vi "Test Case, Table Cell Color.vi"() -> ()   [LabVIEW 2010]
panel:
  in  "dst col":i32=3
  in  "dst row":i32=3
  in  "n rows":i32=5
  in  "error in":errorcluster
  out "error out":errorcluster
  in  "Dst":string[][](table)
  in  "Src":string[][](table)=[["", "", ""], ["", "", ""], ["", "", ""]]
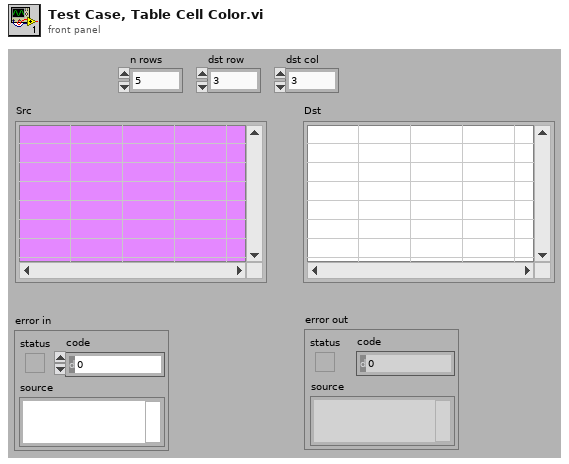
[diagram p1: front panel]
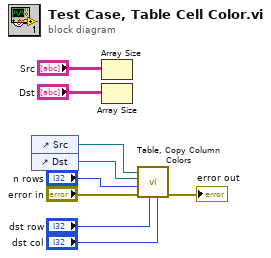
[diagram p0: block diagram]
diagram:
  n1 = control-ref of="Src"() -> (w5:refnum<vi>)
  n2 = control-ref of="Dst"() -> (w6:refnum<vi>)
  n3 = Array Size(array="Src") -> ()  [unwired: 1 out]
  n4 = Array Size(array="Dst") -> ()  [unwired: 1 out]
  n5 = call "Table, Copy Column Colors.vi"("dst col (0)"="dst col", "dst row (0)"="dst row", "error in"="error in", "n rows (1)"="n rows", "Tbl Refnum Dst"=w6, "Tbl Refnum Src"=w5) -> ("error out"=→"error out":errorcluster)  [unwired: 3 in, 2 out]
